vi "tm_setmasterpulse.vi"(8 "error in (no error)":errorcluster, 10 "Parameters":T1={"Mode"=1, "Source"=1, "Interval"=1.0, "Burst"=0} {"Source" items=["External"=1, "Software"=2]; "Mode" items=["Continuous"=1, "Start"=2, "Burst"=3]}, 11 "Handle in":u32) -> (0 "error out":errorcluster, 3 "Handle out":u32)   [LabVIEW 2023]
uses:
  tmcamcon.dll
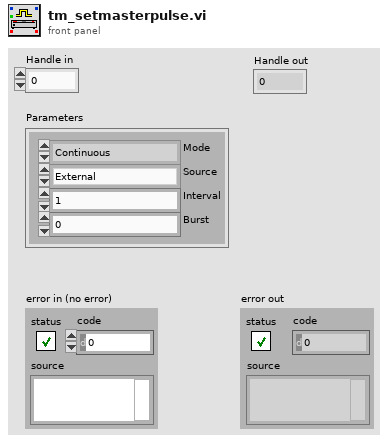
[diagram p1: front panel]
types:
  T1 = cluster{"Mode":u32, "Source":u32, "Interval":dbl, "Burst":u32}
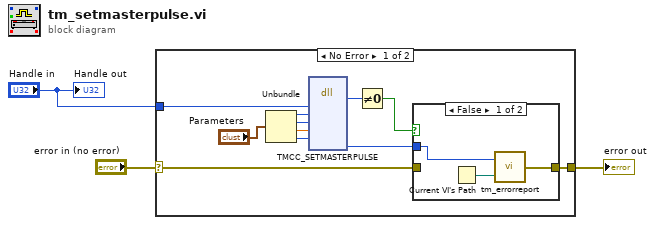
[diagram p0: block diagram]
diagram:
  n1 = case shown="No Error" "error in (no error)" {
    selector: "error in (no error)" -> [w7 w19]
    tunnel: [w4 w19] -> w2
    tunnel: "Handle in" -> [w8 _]
    frame No Error {
      n2 = Unbundle("Parameters") -> ("Mode"=w12:u32, "Source"=w11:u32, "Interval"=w10:dbl, "Burst"=w9:u32)
      n3 = dll-call lib="tmcamcon.dll" fn="TMCC_SETMASTERPULSE"("HDCAM"=w8, "mode"=w12, "source"=w11, "interval"=w10, "bursttimes"=w9) -> ("return type"=w14:u32, "Erval"=w6:i32)  [unwired: 9 in, 2 out]
      n4 = Not Equal To 0?(x=w14) -> (x != 0?=w5:bool)
      n5 = case shown="False" w5 {
        tunnel: w7 -> [_ w18]
        tunnel: [w16 w18] -> w4
        tunnel: w6 -> [w15 _]
        frame False {
          n6 = Current VI's Path() -> (path=w17:path)
          n7 = call "tm_errorreport.vi"("Source"=w17, "Error"=w15) -> ("error out"=w16:errorcluster)
        }
        frame True {
        }
      }
    }
    frame Error {
    }
  }
  "error out" <- w2
  "Handle out" <- "Handle in"
